vi "ActivateAnalogVelocitySettingValue.vi"(4 "error in (no error)":errorcluster, 6 "analog velocity setting":T1, 7 "axis in":cluster{"keyHandle":u32, "nodeId":u16}={"keyHandle"=0, "nodeId"=1}) -> (0 "error out":errorcluster, 3 "axis out":cluster{"keyHandle":u32, "nodeId":u16}={"keyHandle"=0, "nodeId"=1})   [LabVIEW 2010]
doc: "<B>ActivateAnalogVelocitySettingValue</B> configures the selected analog input for analog velocity setpoint."
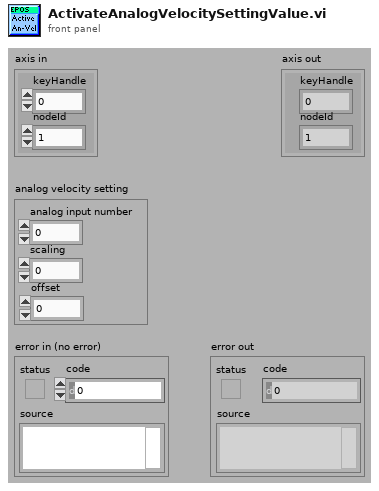
[diagram p1: front panel]
types:
  T1 = cluster{"analog input number":u16, "scaling":sgl, "offset":i32}
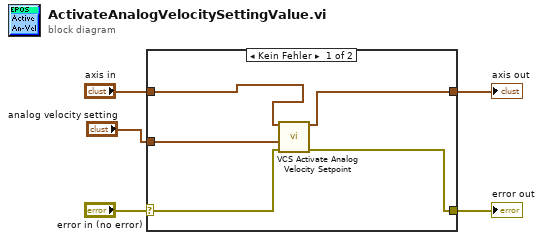
[diagram p0: block diagram]
diagram:
  n1 = case shown="Kein Fehler" "error in (no error)" {
    selector: "error in (no error)" -> [w10 w12]
    tunnel: [w7 w12] -> w4
    tunnel: [w8 w11] -> w3
    tunnel: "axis in" -> [w9 w11]
    tunnel: "analog velocity setting" -> [w6 _]
    frame No Error {
      n2 = call "VCS Activate Analog Velocity Setpoint.vi"("axis in"=w9, "analog velocity setting"=w6, "error in (no error)"=w10) -> ("axis out"=w8:cluster{"keyHandle":u32, "nodeId":u16}, "error out"=w7:errorcluster)  [unwired: 11 in]
    }
    frame Error {
    }
  }
  "error out" <- w4
  "axis out" <- w3
